vi "Get Internal Ignore List.vi"() -> (2 "Success?":bool, 3 "Lower case internal ignores":string[](array[string]))   [LabVIEW 2019, in "Project.Dependencies Finder.lvlib"]
uses:
  Project.Dependencies Finder.lvlib
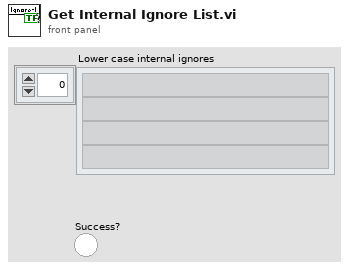
[diagram p1: front panel]
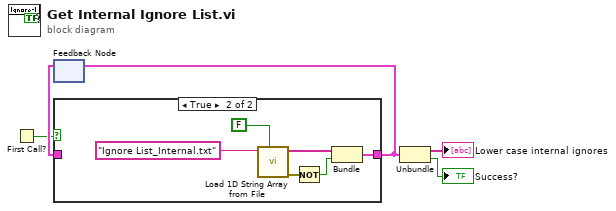
[diagram p0: block diagram]
diagram:
  n1 = First Call?() -> (First Call?: T/F=w1:bool)
  n2 = feedback #1() -> (w2:cluster{"Loaded 1D String Array":string[], bool})  [unwired: 1 in]
  n3 = case shown="True" w1 {
    tunnel: [w6 w7] -> w3
    tunnel: w2 -> [w6 _]
    frame False {
    }
    frame True {
      n4 = call "Load 1D String Array from File.vi"("Remove empty strings?(T)"=FALSE, "File name"="Ignore List_Internal.txt" ("name or relative path")) -> ("error out"=w10:errorcluster, "Loaded 1D String Array"=w11:string[])  [unwired: 8 in]
      n5 = Not(x=w10) -> (.not. x?=w12:bool)
      n6 = Bundle("Loaded 1D String Array"=w11, w12) -> (w7:cluster{"Loaded 1D String Array":string[], bool})  [unwired: 1 in]
    }
  }
  n7 = feedback-in #1(w3) -> ()
  n8 = Unbundle(w3) -> ("Loaded 1D String Array"=→"Lower case internal ignores":string[], →"Success?":bool)
